vi "Add Items.vi"(4 "indent":i32, 6 "Insertion index":i32, 8 "error in (no error)":errorcluster, 10 "Items to Add":refnum<class "BetterItem.lvclass">[](array[class]), 11 "BetterBoxHandle in":refnum<class "BetterBoxHandle.lvclass">) -> (0 "error out":errorcluster, 3 "BetterBoxHandle out":refnum<class "BetterBoxHandle.lvclass">)   [LabVIEW 2020, in "BetterDragAndDrop.lvlib" / "BetterBoxHandle.lvclass"]
uses:
  BetterBoxHandle.lvclass
  C:/DSCE code/Open-source/betterdraganddrop_GIT/Source/Classes/BetterHandle/BetterHandle.lvclass
  BetterTreeItem/BetterItem.lvclass
  BetterHandle/BetterHandle.lvclass/BetterHandle.ctl
  BetterTreeItem/BetterItem.lvclass/BetterItem.ctl
  BetterHandle/BetterHandle.lvclass
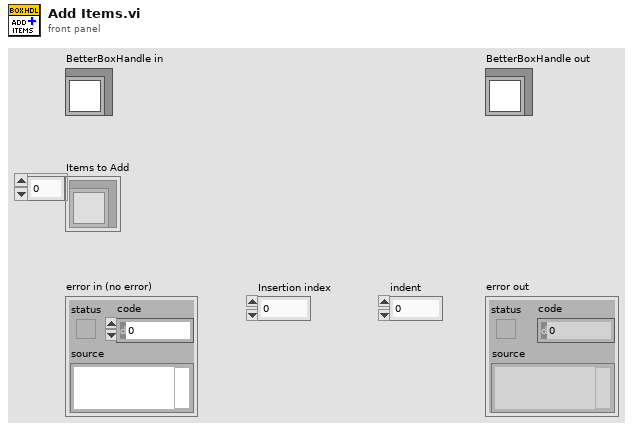
[diagram p1: front panel]
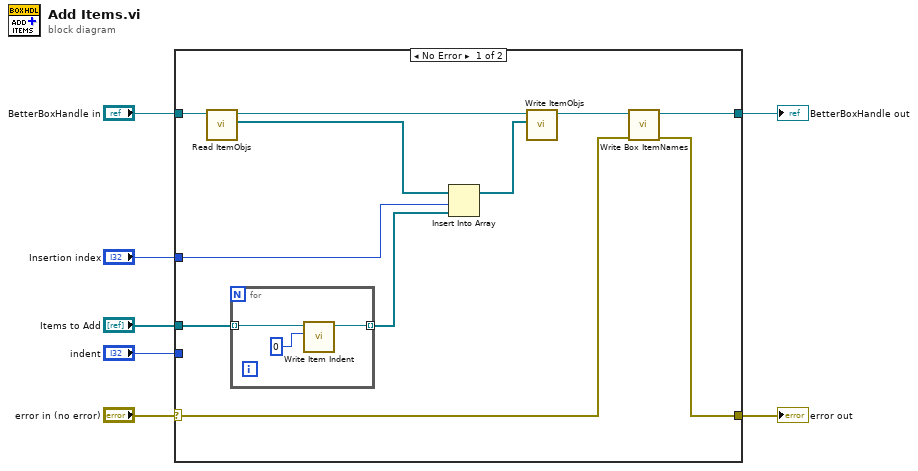
[diagram p0: block diagram]
diagram:
  n1 = case shown="No Error" "error in (no error)" {
    selector: "error in (no error)" -> [w10 w23]
    tunnel: [w9 w23] -> w1
    tunnel: "indent" -> [_ _]
    tunnel: "Insertion index" -> [w18 _]
    tunnel: "BetterBoxHandle in" -> [w17 w22]
    tunnel: [w8 w22] -> w6
    tunnel: "Items to Add" -> [w12 _]
    frame No Error {
      n2 = call "Read ItemObjs.vi"("BetterHandle in"=w17) -> ("ItemObjs"=w16:refnum<class "BetterItem.lvclass">[], "BetterHandle out"=w13:refnum<class "BetterBoxHandle.lvclass">)  [unwired: 9 in]
      n3 = for {
        tunnel: [w19] -> w14 mode=indexing
        tunnel: w12 -> [w21] mode=indexing
        n4 = call "Write Item Indent.vi"("Item Indent"=0, "BetterTreeItem in"=w21) -> ("BetterTreeItem out"=w19:refnum<class "BetterItem.lvclass">)  [unwired: 9 in]
      }
      n5 = Insert Into Array(array=w16, index=w18, new element=w14) -> (w15:refnum<class "BetterItem.lvclass">[])
      n6 = call "Write ItemObjs.vi"("ItemObjs"=w15, "BetterHandle in"=w13) -> ("BetterHandle out"=w11:refnum<class "BetterBoxHandle.lvclass">)  [unwired: 9 in]
      n7 = call-dynamic "Write Box ItemNames.vi"("error in (no error)"=w10, "BetterBoxHandle in"=w11) -> ("error out"=w9:errorcluster, "BetterBoxHandle out"=w8:refnum<class "BetterBoxHandle.lvclass">)  [unwired: 8 in]
    }
    frame Error {
    }
  }
  "error out" <- w1
  "BetterBoxHandle out" <- w6
